vi "SEN_Loop.vi"() -> ()   [LabVIEW 2020, in "PigeonIMU_SEN.lvlib"]
uses:
  PigeonIMU_SEN.lvlib
  <vilib>/Rock Robotics/WPI/ThirdParty/Phoenix-LabVIEW/Pigeon2/controls/CTRE_Phoenix_Pigeon2_Configurables.ctl
  Cluster_CMD_SEN_Data.ctl
  Shared Code/TypeDefs/Cluster_Unity Yaw-Pitch-Roll.ctl
  Shared Code/TypeDefs/Dial_Compase heading unit circle CCW positive.ctl
  Type Defs/Cluster_Yaw Pitch Roll in Deg.ctl
  Type Defs/Cluster_Pigeon Tilt Data.ctl
  Shared Code/TypeDefs/ENUM_Tilt State.ctl
  Shared Code/TypeDefs/Cluster_Tilt Data.ctl
  ENUM_SEN_State.ctl
  <vilib>/Rock Robotics/WPI/ThirdParty/Phoenix-LabVIEW/Pigeon IMU/CTRE_PigeonIMU_DeviceRef.ctl
  <vilib>/Rock Robotics/WPI/ThirdParty/Phoenix-LabVIEW/Pigeon IMU/CTRE_PigeonIMU_ConnectionType.ctl
  Shared Code/TypeDefs/Cluster_Config_PigoenSW Data.ctl
  ENUM_SEN_Action.ctl
  38a3c8f8-8e9e-4176-a30b-59334702453f.vi
  1049c0cb-1755-4509-ba62-f67c8028ea0a.vi
  ca1e8ace-5cb3-4d4b-8a00-bfa7a3df30b2.vi
  2f539002-c075-420f-813a-81d7a1ef4ac8.vi
  38a3c8f8-8e9e-4176-a30b-59334702453f.vi/f38ca901-adc1-4ad8-996e-31aeb746ae36.vi
  38a3c8f8-8e9e-4176-a30b-59334702453f.vi/958b2683-dd4b-41b7-8ed1-41c95f63cef0.vi
  1049c0cb-1755-4509-ba62-f67c8028ea0a.vi/f38ca901-adc1-4ad8-996e-31aeb746ae36.vi
  1049c0cb-1755-4509-ba62-f67c8028ea0a.vi/958b2683-dd4b-41b7-8ed1-41c95f63cef0.vi
  38a3c8f8-8e9e-4176-a30b-59334702453f.vi/f38ca901-adc1-4ad8-996e-31aeb746ae36.vi/1c6bd52c-bbca-4d4a-a290-93ea2703fded.vi
  38a3c8f8-8e9e-4176-a30b-59334702453f.vi/f38ca901-adc1-4ad8-996e-31aeb746ae36.vi/47c2b0d5-b5fa-444e-9535-611565d375db.vi
  1049c0cb-1755-4509-ba62-f67c8028ea0a.vi/f38ca901-adc1-4ad8-996e-31aeb746ae36.vi/1c6bd52c-bbca-4d4a-a290-93ea2703fded.vi
  1049c0cb-1755-4509-ba62-f67c8028ea0a.vi/f38ca901-adc1-4ad8-996e-31aeb746ae36.vi/47c2b0d5-b5fa-444e-9535-611565d375db.vi
  Global_CMD_SEN_Data In.vi
  Utility/Global_STOP.vi
  <vilib>/Utility/Data Type/Get Type Information.vi
  <vilib>/Utility/error.llb/Trim Whitespace.vi
  Shared Code/Utility/RWA/RWA/File/RWA_PC FIle Read String.vi
  Shared Code/Utility/RWA/RWA/Read Write Anything/RWA_File String.vi
  Shared Code/Utility/RWA/RWA/File/RWA_PC File Write String.vi
  Global_SEN_Data Out.vi
  <vilib>/Rock Robotics/WPI/ThirdParty/Phoenix-LabVIEW/Pigeon IMU/CTRE_PigeonIMU_GetRawGyro.vi
  <vilib>/Rock Robotics/WPI/ThirdParty/Phoenix-LabVIEW/Pigeon IMU/CTRE_PigeonIMU_GetFusedHeading.vi
  SwerveOdometry/Global_CMD_SEN_Data In.vi
  SwerveOdometry/Swerve_Odometry_SEN.lvlib
panel:
  in  "Tilt":T1={"Change Threshold (0-1)"=0.01, "Angle Threshold (0-1)"=0.02, "Sample Size"=25}
  out "Tilt Data":T2
  out "Yaw Pitch Roll Deg":T4
  out "Pigeon Running":bool
  out "YawPitchRoll":T5 {"Roll" scale format="%.3f"; "Pitch" scale format="%.3f"; "Yaw" scale format="%.3f"}
  in  "CMD_SEN_Pigeon_Data":T7
  in  "Set Values":bool
  in  "Pigeon2 Config":T8
  out "Pigeon Ready":bool
  out "Pigeon Enabled":bool
  out "Cycle Time (S)":dbl format="%.3g"
  # "Yaw Angle needed to reach the current orientation in degrees"
  # "Configures the mounting pose of the Pigeon2\nThis is the yaw-pitch-roll teh Pigeon2 underwent to get to its current orientation,\n referenced from the robot's point of view\nThis is only necessary if the Pigeon2 is mounted at an exotic angle near the gimbal lock point or not forward.\nIf the pigeon is relatively flat and pointed forward, this is not needed"
  # "Pitch Angle needed to reach the current orientation in degrees"
  # "Roll Angle needed to reach the current orientation in degrees"
  # "Disables the temperature compensation\nfrom the Pigeon2. It is recommended that\nthis remains false"
  # "Disables the no-motion calibration from the\nPigeon2. It is recommended that this \nremains false"
  # "Enables the compass for Pigeon2\nThis is not recommended for any indoor robotics"
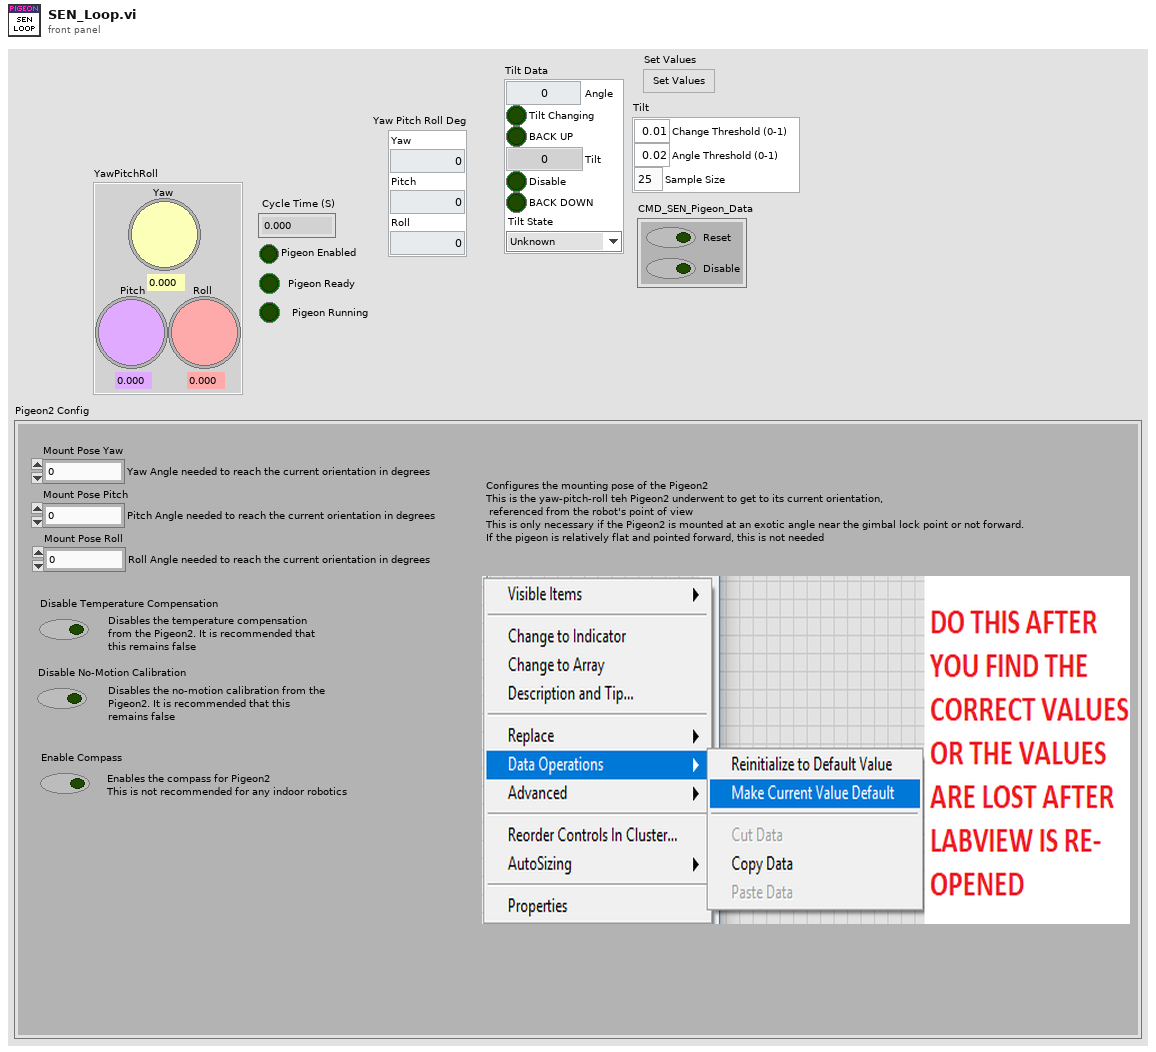
[diagram p1: front panel]
types:
  T1 = typedef "Cluster_Tilt Data.ctl" = cluster{"Change Threshold (0-1)":dbl, "Angle Threshold (0-1)":dbl, "Sample Size":i32}
  T2 = typedef "Cluster_Pigeon Tilt Data.ctl" = cluster{"Angle":dbl, "Tilt Changing":bool, "BACK UP":bool, "Tilt":dbl, "Disable":bool, "BACK DOWN":bool, "Tilt State":T3}
  T3 = typedef "ENUM_Tilt State.ctl" = enum16{"Unknown", "Level", "Angle UP from Level", "Level from Angle Up", "Angle Down from Level", "Level from Angle Down"}
  T4 = typedef "Cluster_Yaw Pitch Roll in Deg.ctl" = cluster{"Yaw":dbl, "Pitch":dbl, "Roll":dbl}
  T5 = typedef "Cluster_Unity Yaw-Pitch-Roll.ctl" = cluster{"Yaw":T6, "Pitch":T6, "Roll":T6}
  T6 = typedef "Dial_Compase heading unit circle CCW positive.ctl" = dbl
  T7 = typedef "PigeonIMU_SEN.lvlib/Cluster_CMD_SEN_Data.ctl" = cluster{"Reset":bool, "Disable":bool}
  T8 = typedef "CTRE_Phoenix_Pigeon2_Configurables.ctl" = cluster{"Mount Pose Yaw":dbl, "Mount Pose Pitch":dbl, "Mount Pose Roll":dbl, "Disable Temperature Compensation":bool, "Disable No-Motion Calibration":bool, "Enable Compass":bool}
  T9 = typedef "Cluster_Config_PigoenSW Data.ctl" = cluster{"PigeonSW Ver":u64, "Tilt":T1}
  T10 = cluster{"Heading":dbl, "Valid?":bool, "Fusing?":bool}
  T11 = typedef "CTRE_PigeonIMU_DeviceRef.ctl" = cluster{"DeviceStatus":errorcluster, "Device Number":u8, "Type":T12, "Device ID":u32, "Handle":u64, "UsageFrame":u32, "Library Path":path}
  T12 = typedef "CTRE_PigeonIMU_ConnectionType.ctl" = u32
  T13 = typedef "PigeonIMU_SEN.lvlib/ENUM_SEN_State.ctl" = enum16{"Starting", "Reseting", "Enableing", "Disabeling", "Shutting Down"}
  T14 = cluster{"PigeonIMUDevRef":T11, "State":T13, "Previous State":T13, "Current Time":timestamp, "Previous Time":timestamp, "Start Time":timestamp, "Target Time (ms)":u32, "Cycle Time(S)":dbl, "Reset":bool, "Yaw Pitch Roll Unit":T5, "Fused Heading":cluster{"Heading":dbl, "Valid?":bool, "Fusing?":bool}, "IMU Ready":bool, "Swing Threshold":dbl, "Swing Array Size":i32, "CMD_SEN_Pigeon_Data":T7, "Tilt Data":T2, "Yaw Pitch Roll Deg":T4, "Pigeon Running":bool, "Pigeon Config":T9, "Team Files Folder":path, "Offset Values":cluster{"Y":dbl, "X":dbl, "Degrees":dbl}}
  T15 = typedef "PigeonIMU_SEN.lvlib/ENUM_SEN_Action.ctl" = enum16{"No Action", "Reset Time", "Zero Heading", "Read Heading", "Read Raw ", "Configure IMU", "Check IMU Reset", "Set Enable Cycle Time", "Set Disable Cycle Time", "Config From FP", "Config Save to File", "Config Read from File"}
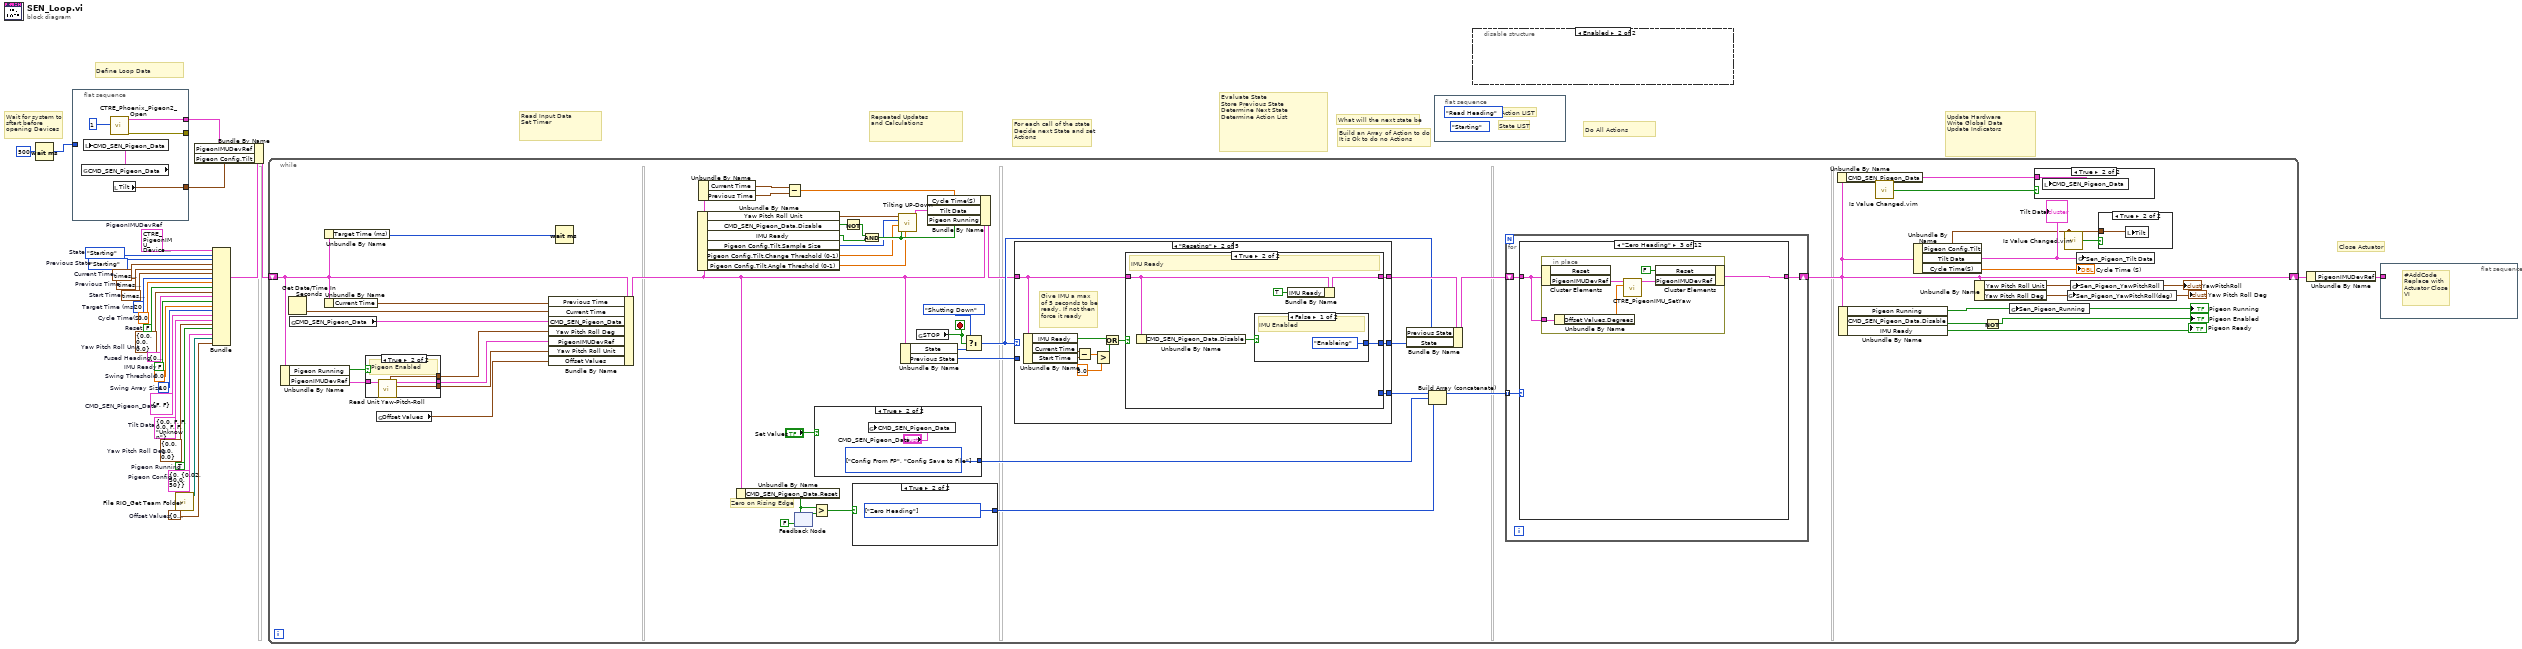
[diagram p0: block diagram]
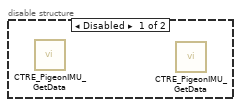
[diagram p2: hidden frame]
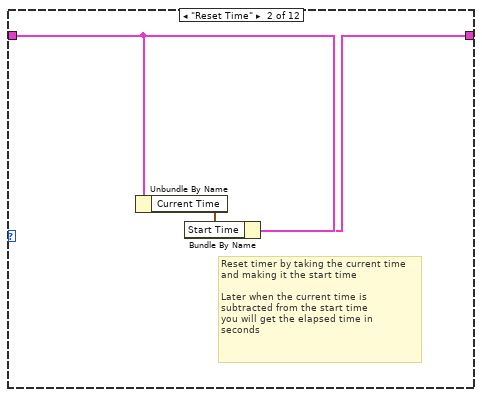
[diagram p9: hidden frame]
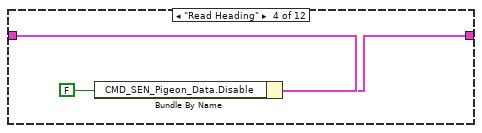
[diagram p10: hidden frame]
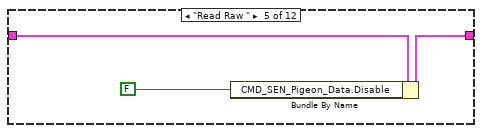
[diagram p11: hidden frame]
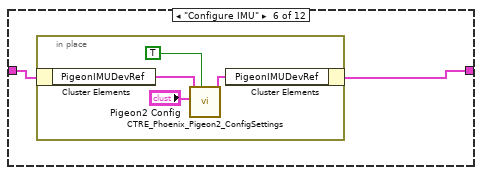
[diagram p12: hidden frame]
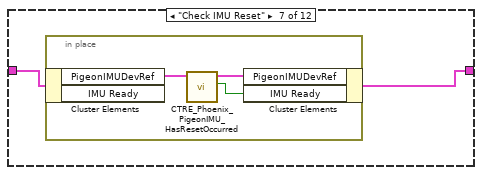
[diagram p13: hidden frame]
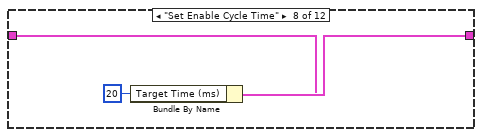
[diagram p14: hidden frame]
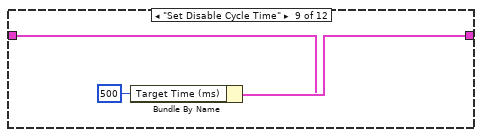
[diagram p15: hidden frame]
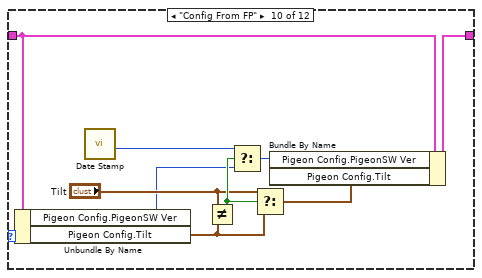
[diagram p16: hidden frame]
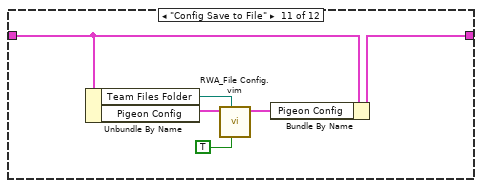
[diagram p17: hidden frame]
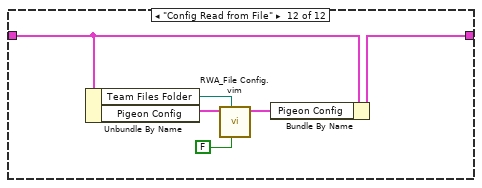
[diagram p18: hidden frame]
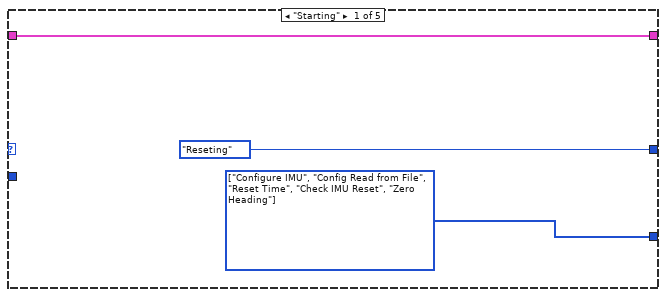
[diagram p19: hidden frame]
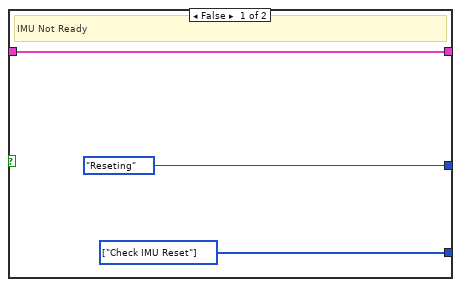
[diagram p20: hidden frame]
diagram:
  w1 = cluster{"Y":dbl, "X":dbl, "Degrees":dbl} {"Y"=0.0, "X"=0.0, "Degrees"=0.0}  # Offset Values
  w4 = T9 {"PigeonSW Ver"=0, "Tilt"={"Change Threshold (0-1)"=0.02, "Angle Threshold (0-1)"=50.0, "Sample Size"=50}}  # Pigeon Config
  w5 = TRUE  # Pigeon Running
  w6 = T4 {"Yaw"=0.0, "Pitch"=0.0, "Roll"=0.0}  # Yaw Pitch Roll Deg
  w7 = T2 {"Angle"=0.0, "Tilt Changing"=FALSE, "BACK UP"=FALSE, "Tilt"=0.0, "Disable"=FALSE, "BACK DOWN"=FALSE, "Tilt State"=enum."Unknown"}  # Tilt Data
  w8 = T5 {"Yaw"=0.0, "Pitch"=0.0, "Roll"=0.0}  # Yaw Pitch Roll Unit
  w9 = T7 {"Reset"=FALSE, "Disable"=FALSE}  # CMD_SEN_Pigeon_Data
  w10 = 10  # Swing Array Size
  w11 = 0.0  # Swing Threshold
  w12 = FALSE  # IMU Ready
  w13 = T10 {"Heading"=0.0, "Valid?"=FALSE, "Fusing?"=FALSE}  # Fused Heading
  w14 = T11 {"DeviceStatus"={"status"=FALSE, "code"=0, "source"=""}, "Device Number"=0, "Type"=352321536, "Device ID"=0, "Handle"=0, "UsageFrame"=0, "Library Path"=path ""}  # PigeonIMUDevRef
  w22 = 0.0  # Cycle Time(S)
  w23 = ENUM_SEN_State."Starting"  # Previous State
  w24 = timestamp(0 s since 1904-01-01)  # Previous Time
  w25 = u32 20  # Target Time (ms)
  w26 = FALSE  # Reset
  w27 = timestamp(0 s since 1904-01-01)  # Start Time
  w28 = timestamp(0 s since 1904-01-01)  # Current Time
  w29 = ENUM_SEN_State."Starting"  # State
  # "Wait for system to\nsftart before\nopening Devices"
  # "Build an Array of Action to do\nIt is Ok to do no Actions"
  # "What will the next state be"
  # "For each call of the state\nDecide next State and set\nActions"
  # "Close Actuator"
  # "Define Loop Data"
  # "Repeated Updates\nand Calculations"
  # "Read Input Data\nSet Timer"
  # "Evaluate State\nStore Previous State\nDetermine Next State\nDetermine Action List"
  # "Do All Actions"
  # "Update Hardware\nWrite Global Data\nUpdate Indicators"
  n1 = Wait (ms)(milliseconds to wait=u32 500) -> (millisecond timer value=w15:u32)
  n2 = flat-sequence {
    tunnel: [w34] -> w17
    tunnel: w15 -> [_]
    tunnel: [w31] -> _
    tunnel: [w30] -> w2
    frame #0 {
      n3 = global read "Global_CMD_SEN_Data In.vi" "CMD_SEN_Pigeon_Data"() -> (w32:T7)
      n4 = local write "CMD_SEN_Pigeon_Data"(w32) -> ()
      n5 = call <vilib>:"CTRE_Phoenix_Pigeon2_Open.vi"("Device Number"=u8 1) -> ("error out"=w31:errorcluster, "PigeonIMUDevRef"=w34:T11)  [unwired: 9 in]
      n6 = local read "Tilt"() -> (w30:T1)
    }
  }
  n7 = call "File RIO_Get Team Folder.vi"() -> ("Team Files Folder"=w3:path)  [unwired: 10 in, 1 out]
  n8 = Bundle("PigeonIMUDevRef"=w14, "State"=w29, "Previous State"=w23, "Current Time"=w28, "Previous Time"=w24, "Start Time"=w27, "Target Time (ms)"=w25, "Cycle Time(S)"=w22, "Reset"=w26, "Yaw Pitch Roll Unit"=w8, "Fused Heading"=w13, "IMU Ready"=w12, "Swing Threshold"=w11, "Swing Array Size"=w10, "CMD_SEN_Pigeon_Data"=w9, "Tilt Data"=w7, "Yaw Pitch Roll Deg"=w6, "Pigeon Running"=w5, "Pigeon Config"=w4, "Team Files Folder"=w3, "Offset Values"=w1) -> (w19:T14)  [unwired: 1 in]
  n9 = Bundle By Name(cluster=w19, "PigeonIMUDevRef"=w17, "Pigeon Config.Tilt"=w2) -> (w18:T14)
  n10 = while {
    shift-right: [w57] -> w20
    shift-left: w18 -> [w47]
    stop <- w85 stop-if-true
    # "Zero on Rising Edge"
    n11 = Unbundle By Name(w47) -> ("Pigeon Running"=w46:bool, "PigeonIMUDevRef"=w48:T11)
    n12 = Get Date/Time In Seconds() -> (seconds since 1Jan1904=w89:timestamp)
    n13 = global read "Global_CMD_SEN_Data In.vi" "CMD_SEN_Pigeon_Data"() -> (w61:T7)
    n14 = Unbundle By Name(w47) -> ("Target Time (ms)"=w82:u32)
    n15 = Unbundle By Name(w47) -> ("Current Time"=w81:timestamp)
    n16 = case shown="True" w46 {
      tunnel: w48 -> [w91 w92]
      tunnel: [w91 w95] -> w44
      tunnel: [_ w94] -> w43
      tunnel: [_ w93] -> w45
      frame False {
        # "Pigeon Disabled"
      }
      frame True {
        # "Pigeon Enabled"
        n17 = call "Read Unit Yaw-Pitch-Roll.vi"("PigeonIMUDevRef"=w92) -> ("Unit Yaw-Pitch-Roll Out"=w94:T5, "PigeonIMUDevRef Out"=w95:T11, "Yaw Pitch Roll Out"=w93:T4)  [unwired: 8 in]
      }
    }
    n18 = global read "Global_CMD_SEN_Data In.vi" "Offset Values"() -> (w35:cluster{"Y":dbl, "X":dbl, "Degrees":dbl})
    n19 = Bundle By Name(cluster=w47, "Previous Time"=w81, "Current Time"=w89, "CMD_SEN_Pigeon_Data"=w61, "Yaw Pitch Roll Deg"=w45, "PigeonIMUDevRef"=w44, "Yaw Pitch Roll Unit"=w43, "Offset Values"=w35) -> (w67:T14)
    n20 = Wait (ms)(milliseconds to wait=w82) -> ()  [unwired: 1 out]
    n21 = Unbundle By Name(w67) -> ("Yaw Pitch Roll Unit"=w66:T5, "CMD_SEN_Pigeon_Data.Disable"=w54:bool, "IMU Ready"=w56:bool, "Pigeon Config.Tilt.Sample Size"=w42:i32, "Pigeon Config.Tilt.Change Threshold (0-1)"=w37:dbl, "Pigeon Config.Tilt.Angle Threshold (0-1)"=w36:dbl)
    n22 = Unbundle By Name(w67) -> ("Current Time"=w68:timestamp, "Previous Time"=w78:timestamp)
    n23 = Unbundle By Name(w67) -> ("CMD_SEN_Pigeon_Data.Reset"=w71:bool)
    n24 = Subtract(x=w68, y=w78) -> (x-y=w76:dbl)
    n25 = feedback-in #1(w71) -> ()
    n26 = feedback #1(FALSE ("CMD_SEN_Pigeon_Reset")) -> (w72:bool)
    n27 = Greater?(x=w71, y=w72) -> (0:w70:bool)
    n28 = case shown="True" "Set Values" {
      tunnel: [_ w97] -> w38
      frame False {
      }
      frame True {
        w97 = T15[] [enum."Config From FP", enum."Config Save to File"] items=["No Action", "Reset Time", "Zero Heading", "Read Heading", "Read Raw ", "Configure IMU", "Check IMU Reset", "Set Enable Cycle Time", "Set Disable Cycle Time", "Config From FP", "Config Save to File", "Config Read from File"] ("Actions")
        n29 = global write "Global_CMD_SEN_Data In.vi" "CMD_SEN_Pigeon_Data"("CMD_SEN_Pigeon_Data") -> ()
      }
    }
    n30 = Not(x=w54) -> (.not. x?=w55:bool)
    n31 = case shown="True" w70 {
      tunnel: [_ w99] -> w39
      frame False {
      }
      frame True {
        w99 = T15[] [enum."Zero Heading"] items=["No Action", "Reset Time", "Zero Heading", "Read Heading", "Read Raw ", "Configure IMU", "Check IMU Reset", "Set Enable Cycle Time", "Set Disable Cycle Time", "Config From FP", "Config Save to File", "Config Read from File"] ("Actions")
      }
    }
    n32 = And(x=w55, y=w56) -> (x .and. y?=w53:bool)
    n33 = call "Tilting UP-Down.vi"("Angle Threshold (0-1)"=w36, "Pigeon Running"=w53, "Change Threshold (0-1)"=w37, "Tilt Detect Sample Size"=w42, "YawPitchRoll"=w66) -> ("Tilt Data"=w60:T2)  [unwired: 6 in]
    n34 = Unbundle By Name(w67) -> ("State"=w83:T13, "Previous State"=w80:T13)
    n35 = global read "Global_STOP.vi" "STOP"() -> (w85:bool)
    n36 = Bundle By Name(cluster=w67, "Cycle Time(S)"=w76, "Tilt Data"=w60, "Pigeon Running"=w53) -> (w77:T14)
    n37 = Select(t=ENUM_SEN_State."Shutting Down" ("State"), s=w85, f=w83) -> (s? t:f=w79:T13)
    n38 = case shown="\"Reseting\"" w79 {
      tunnel: w77 -> [w160 w170 w185 w200 w213]
      tunnel: [w160 w169 w184 w199 w213] -> w87
      tunnel: [ENUM_SEN_State."Reseting" ("State") w168 w183 w198 ENUM_SEN_State."Shutting Down" ("State")] -> w86
      tunnel: [w158 w167 w182 w197 _] -> w75
      tunnel: w80 -> [_ _ _ _ _]
      frame "Starting" {
        w158 = T15[] [enum."Configure IMU", enum."Config Read from File", enum."Reset Time", enum."Check IMU Reset", enum."Zero Heading"] items=["No Action", "Reset Time", "Zero Heading", "Read Heading", "Read Raw ", "Configure IMU", "Check IMU Reset", "Set Enable Cycle Time", "Set Disable Cycle Time", "Config From FP", "Config Save to File", "Config Read from File"] ("Actions")
      }
      frame "Reseting" {
        # "Give IMU a max\nof 5 seconds to be\nready. If not then\nforce it ready"
        n39 = Unbundle By Name(w170) -> ("IMU Ready"=w171:bool, "Current Time"=w166:timestamp, "Start Time"=w165:timestamp)
        n40 = Subtract(x=w166, y=w165) -> (x-y=w164:dbl)
        n41 = Greater?(x=w164, y=5.0) -> (0:w161:bool)
        n42 = Or(x=w171, y=w161) -> (x .or. y?=w162:bool)
        n43 = case shown="True" w162 {
          tunnel: w170 -> [w172 w176]
          tunnel: [w172 w177] -> w169
          tunnel: [ENUM_SEN_State."Reseting" ("State") w179] -> w168
          tunnel: [w173 _] -> w167
          frame False {
            w173 = T15[] [enum."Check IMU Reset"] items=["No Action", "Reset Time", "Zero Heading", "Read Heading", "Read Raw ", "Configure IMU", "Check IMU Reset", "Set Enable Cycle Time", "Set Disable Cycle Time", "Config From FP", "Config Save to File", "Config Read from File"] ("Actions")
            # "IMU Not Ready"
          }
          frame True {
            # "IMU Ready"
            n44 = Unbundle By Name(w176) -> ("CMD_SEN_Pigeon_Data.Disable"=w178:bool)
            n45 = case shown="False" w178 {
              tunnel: [ENUM_SEN_State."Enableing" ("State") ENUM_SEN_State."Disabeling" ("State")] -> w179
              frame False {
                # "IMU Enabled"
              }
              frame True {
                # "IMU Disabled"
              }
            }
            n46 = Bundle By Name(cluster=w176, "IMU Ready"=TRUE) -> (w177:T14)
          }
        }
      }
      frame "Enableing" {
        n47 = Unbundle By Name(w185) -> ("IMU Ready"=w186:bool)
        n48 = case shown="True" w186 {
          tunnel: w185 -> [w187 w192]
          tunnel: [w187 w192] -> w184
          tunnel: [ENUM_SEN_State."Reseting" ("State") w193] -> w183
          tunnel: [w188 w190] -> w182
          frame False {
            w188 = T15[] [enum."Check IMU Reset"] items=["No Action", "Reset Time", "Zero Heading", "Read Heading", "Read Raw ", "Configure IMU", "Check IMU Reset", "Set Enable Cycle Time", "Set Disable Cycle Time", "Config From FP", "Config Save to File", "Config Read from File"] ("Actions")
            # "IMU Not Ready"
          }
          frame True {
            # "IMU Ready"
            n49 = Unbundle By Name(w192) -> ("CMD_SEN_Pigeon_Data.Disable"=w191:bool)
            n50 = case shown="False" w191 {
              tunnel: [ENUM_SEN_State."Enableing" ("State") ENUM_SEN_State."Disabeling" ("State")] -> w193
              tunnel: [w194 _] -> w190
              frame False {
                w194 = T15[] [enum."Set Enable Cycle Time"] items=["No Action", "Reset Time", "Zero Heading", "Read Heading", "Read Raw ", "Configure IMU", "Check IMU Reset", "Set Enable Cycle Time", "Set Disable Cycle Time", "Config From FP", "Config Save to File", "Config Read from File"] ("Actions")
                # "IMU Enabled"
              }
              frame True {
                # "IMU Disabled"
              }
            }
          }
        }
      }
      frame "Disabeling" {
        n51 = Unbundle By Name(w200) -> ("IMU Ready"=w201:bool)
        n52 = case shown="True" w201 {
          tunnel: w200 -> [w202 w207]
          tunnel: [w202 w207] -> w199
          tunnel: [ENUM_SEN_State."Reseting" ("State") w208] -> w198
          tunnel: [w203 w205] -> w197
          frame False {
            w203 = T15[] [enum."Check IMU Reset"] items=["No Action", "Reset Time", "Zero Heading", "Read Heading", "Read Raw ", "Configure IMU", "Check IMU Reset", "Set Enable Cycle Time", "Set Disable Cycle Time", "Config From FP", "Config Save to File", "Config Read from File"] ("Actions")
            # "IMU Not Ready"
          }
          frame True {
            # "IMU Ready"
            n53 = Unbundle By Name(w207) -> ("CMD_SEN_Pigeon_Data.Disable"=w206:bool)
            n54 = case shown="True" w206 {
              tunnel: [ENUM_SEN_State."Enableing" ("State") ENUM_SEN_State."Disabeling" ("State")] -> w208
              tunnel: [_ w210] -> w205
              frame False {
                # "IMU Enabled"
              }
              frame True {
                w210 = T15[] [enum."Set Disable Cycle Time"] items=["No Action", "Reset Time", "Zero Heading", "Read Heading", "Read Raw ", "Configure IMU", "Check IMU Reset", "Set Enable Cycle Time", "Set Disable Cycle Time", "Config From FP", "Config Save to File", "Config Read from File"] ("Actions")
                # "IMU Disabled"
              }
            }
          }
        }
      }
      frame "Shutting Down" {
      }
    }
    n55 = Bundle By Name(cluster=w87, "Previous State"=w79, "State"=w86) -> (w88:T14)
    n56 = Build Array (concatenate)(w75, w38, w39) -> (w69:T15[])
    n57 = for {
      tunnel: w69 -> [w102] mode=indexing
      shift-right: [w101] -> w57
      shift-left: w88 -> [w100]
      n58 = case shown="\"Zero Heading\"" w102 {
        tunnel: w100 -> [w103 w106 w107 w116 w119 w121 w127 w132 w135 w137 w147 w153]
        tunnel: [w103 w105 w108 w115 w118 w120 w126 w133 w136 w138 w148 w154] -> w101
        frame "No Action" {
        }
        frame "Reset Time" {
          # "Reset timer by taking the current time\nand making it the start time\n\nLater when the current time is \nsubtracted from the start time\nyou will get the elapsed time in \nseconds"
          n59 = Unbundle By Name(w106) -> ("Current Time"=w104:timestamp)
          n60 = Bundle By Name(cluster=w106, "Start Time"=w104) -> (w105:T14)
        }
        frame "Zero Heading" {
          n61 = in-place {
            in-place-border: w107 -> [w110]
            n62 = in-place-cluster #2(w107) -> ("PigeonIMUDevRef"=w113:T11)  [unwired: 1 out]
            n63 = Unbundle By Name(w110) -> ("Offset Values.Degrees"=w109:dbl)
            n64 = call <vilib>:"CTRE_PigeonIMU_SetYaw.vi"("Value"=w109, "PigeonIMUDevRef"=w113) -> ("PigeonIMUDevRef"=w112:T11)  [unwired: 8 in, 1 out]
            n65 = in-place-cluster #2("Reset"=FALSE, "PigeonIMUDevRef"=w112) -> (w108:T14)
          }
        }
        frame "Read Heading" {
          n66 = Bundle By Name(cluster=w116, "CMD_SEN_Pigeon_Data.Disable"=FALSE ("Read Enable")) -> (w115:T14)
        }
        frame "Read Raw " {
          n67 = Bundle By Name(cluster=w119, "CMD_SEN_Pigeon_Data.Disable"=FALSE ("Read Enable")) -> (w118:T14)
        }
        frame "Configure IMU" {
          n68 = in-place {
            n69 = in-place-cluster #3(w121) -> ("PigeonIMUDevRef"=w125:T11)
            n70 = call <vilib>:"CTRE_Phoenix_Pigeon2_ConfigSettings.vi"("Force Write"=TRUE, "Pigeon2 Configurables"="Pigeon2 Config", "PigeonIMUDevRef 2"=w125) -> ("PigeonIMUDevRef"=w124:T11)  [unwired: 7 in, 1 out]
            n71 = in-place-cluster #3("PigeonIMUDevRef"=w124) -> (w120:T14)
          }
        }
        frame "Check IMU Reset" {
          n72 = in-place {
            n73 = in-place-cluster #4(w127) -> ("PigeonIMUDevRef"=w130:T11)  [unwired: 1 out]
            n74 = call <vilib>:"CTRE_Phoenix_PigeonIMU_HasResetOccurred.vi"("CTRE_PigeonIMU_DeviceRef"=w130) -> ("Has Reset Occurred?"=w128:bool, "CTRE_PigeonIMU_DeviceRef"=w129:T11)  [unwired: 8 in, 1 out]
            n75 = in-place-cluster #4("PigeonIMUDevRef"=w129, "IMU Ready"=w128) -> (w126:T14)
          }
        }
        frame "Set Enable Cycle Time" {
          n76 = Bundle By Name(cluster=w132, "Target Time (ms)"=u32 20) -> (w133:T14)
        }
        frame "Set Disable Cycle Time" {
          n77 = Bundle By Name(cluster=w135, "Target Time (ms)"=u32 500) -> (w136:T14)
        }
        frame "Config From FP" {
          n78 = Unbundle By Name(w137) -> ("Pigeon Config.PigeonSW Ver"=w139:u64, "Pigeon Config.Tilt"=w140:T1)
          n79 = call "Date Stamp.vi"() -> ("U64 Out"=w144:u64)  [unwired: 6 in, 1 out]
          n80 = Not Equal?(x="Tilt", y=w140) -> (x != y?=w145:bool)
          n81 = Select(t=w144, s=w145, f=w139) -> (s? t:f=w143:u64)
          n82 = Select(t="Tilt", s=w145, f=w140) -> (s? t:f=w141:T1)
          n83 = Bundle By Name(cluster=w137, "Pigeon Config.PigeonSW Ver"=w143, "Pigeon Config.Tilt"=w141) -> (w138:T14)
        }
        frame "Config Save to File" {
          n84 = Unbundle By Name(w147) -> ("Team Files Folder"=w150:path, "Pigeon Config"=w151:T9)
          n85 = call "RWA_File Config.vim"("Read(f) Write(t)"=TRUE, "Target Folder Folder"=w150, "Any Config"=w151) -> ("Any Config Out"=w149:T9)  [unwired: 4 in, 4 out]
          n86 = Bundle By Name(cluster=w147, "Pigeon Config"=w149) -> (w148:T14)
        }
        frame "Config Read from File" {
          n87 = Unbundle By Name(w153) -> ("Team Files Folder"=w156:path, "Pigeon Config"=w157:T9)
          n88 = call "RWA_File Config.vim"("Read(f) Write(t)"=FALSE, "Target Folder Folder"=w156, "Any Config"=w157) -> ("Any Config Out"=w155:T9)  [unwired: 4 in, 4 out]
          n89 = Bundle By Name(cluster=w153, "Pigeon Config"=w155) -> (w154:T14)
        }
      }
    }
    n90 = Unbundle By Name(w57) -> ("CMD_SEN_Pigeon_Data"=w63:T7)
    n91 = Unbundle By Name(w57) -> ("Pigeon Running"=w52:bool, "CMD_SEN_Pigeon_Data.Disable"=w51:bool, "IMU Ready"=→"Pigeon Ready":bool)
    "Pigeon Running" <- w52
    n92 = call "Is Value Changed.vim"("value"=w63) -> ("changed or first call?"=w64:bool)
    n93 = Unbundle By Name(w57) -> ("Pigeon Config.Tilt"=w41:T1, "Tilt Data"=w65:T2, "Cycle Time(S)"=→"Cycle Time (S)":dbl)
    "Tilt Data" <- w65
    n94 = Unbundle By Name(w57) -> ("Yaw Pitch Roll Unit"=w59:T5, "Yaw Pitch Roll Deg"=w58:T4)
    "YawPitchRoll" <- w59
    "Yaw Pitch Roll Deg" <- w58
    n95 = Not(x=w51) -> (.not. x?=→"Pigeon Enabled":bool)
    n96 = global write "Global_SEN_Data Out.vi" "Sen_Pigeon_Running"(w52) -> ()
    n97 = case shown="True" w64 {
      tunnel: w63 -> [_ w96]
      frame False {
      }
      frame True {
        n98 = local write "CMD_SEN_Pigeon_Data"(w96) -> ()
      }
    }
    n99 = call "Is Value Changed.vim"("value"=w41) -> ("changed or first call?"=w40:bool)
    n100 = global write "Global_SEN_Data Out.vi" "Sen_Pigeon_YawPitchRoll(deg)"(w58) -> ()
    n101 = global write "Global_SEN_Data Out.vi" "Sen_Pigeon_YawPitchRoll"(w59) -> ()
    n102 = global write "Global_SEN_Data Out.vi" "Sen_Pigeon_Tilt Data"(w65) -> ()
    n103 = case shown="True" w40 {
      tunnel: w41 -> [_ w90]
      frame False {
      }
      frame True {
        n104 = local write "Tilt"(w90) -> ()
      }
    }
  }
  n105 = flat-sequence {
    frame #0 {
      (unwired) ENUM_SEN_State."Starting" ("State")
      (unwired) ENUM_SEN_Action."Read Heading" ("Action")
      # "State LIST"
      # "Action LIST"
    }
  }
  n106 = disable-structure shown="Enabled" {
    frame Disabled {
      n107 = call-poly <vilib>:"CTRE_PigeonIMU_GetData.vi"() -> ()  [unwired: 9 in, 3 out]
      n108 = call-poly <vilib>:"CTRE_PigeonIMU_GetData.vi"() -> ()  [unwired: 9 in, 3 out]
    }
    frame Enabled {
    }
  }
  n109 = Unbundle By Name(w20) -> ("PigeonIMUDevRef"=w21:T11)
  n110 = flat-sequence {
    tunnel: w21 -> [_]
    frame #0 {
      # "#AddCode\nReplace with \nActuator Close\nVI"
    }
  }
